vi "LV Dev Doc - Instantiate with Ref.vi"(0 "VI Refnum":refnum<vi>, 11 "error in (no error)":errorcluster) -> (4 "LV DEV":refnum<class "LV DEV.lvclass">, 15 "error out":errorcluster)   [LabVIEW 2016, in "LV DEV.lvclass"]
uses:
  LV DEV.lvclass
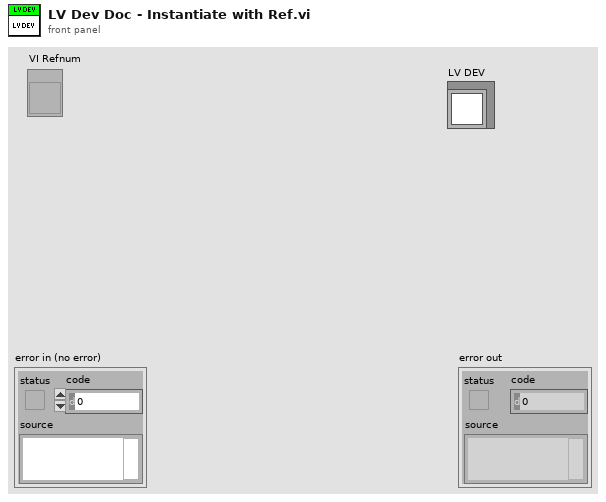
[diagram p1: front panel]
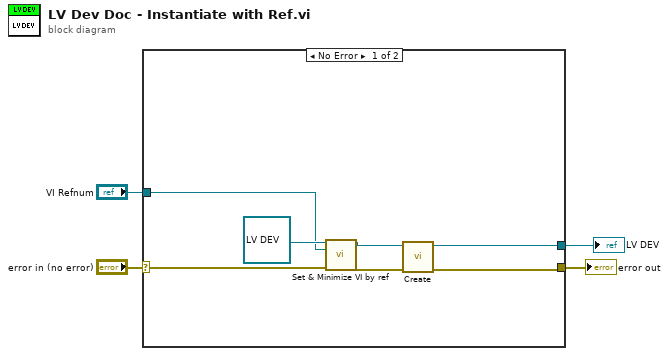
[diagram p0: block diagram]
diagram:
  n1 = case shown="No Error" "error in (no error)" {
    selector: "error in (no error)" -> [w9 w12]
    tunnel: [w11 w12] -> w3
    tunnel: [w10 _] -> w1
    tunnel: "VI Refnum" -> [w5 _]
    frame No Error {
      n2 = call "Set & Minimize VI by ref.vi"("LV DEV.lvclass"=refnum<class "LV DEV.lvclass"> refnum ("LV DEV"), "VI Refnum"=w5, "Error in"=w9) -> ("LV DEV.lvclass"=w7:refnum<class "LV DEV.lvclass">, "Error Out"=w6:errorcluster)  [unwired: 11 in]
      n3 = call-dynamic "Create.vi"("error in (no error)"=w6, "Document in"=w7) -> ("error out"=w11:errorcluster, "Document out"=w10:refnum<class "LV DEV.lvclass">)  [unwired: 8 in]
    }
    frame Error {
    }
  }
  "error out" <- w3
  "LV DEV" <- w1
